vi "NF WF1973_74 SEQ Cst.vi"(8 "error in (no error)":errorcluster caption="Error IN", 10 "Ch(Ch1)":bool, 11 "VISAsession":refnum<visa-resource-name>) -> (0 "error out":errorcluster caption="Error OUT", 2 "Query Step":i32, 3 "CopyVISAsession":refnum<visa-resource-name>)   [LabVIEW 2010]
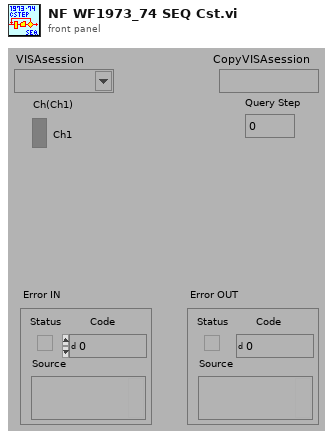
[diagram p1: front panel]
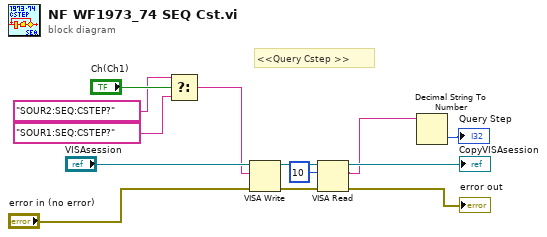
[diagram p0: block diagram]
diagram:
  # "<<Query Cstep >>"
  n1 = Select(t="SOUR2:SEQ:CSTEP?" ("文字列"), s="Ch(Ch1)", f="SOUR1:SEQ:CSTEP?" ("文字列")) -> (s? t:f=w3:string)
  n2 = VISA Write(VISA resource name="VISAsession", write buffer=w3, error in (no error)="error in (no error)") -> (VISA resource name out=w8:refnum<visa-resource-name>, error out=w9:errorcluster)  [unwired: 1 out]
  n3 = VISA Read(VISA resource name=w8, byte count=u32 10 ("バイトカウント（0）"), error in (no error)=w9) -> (VISA resource name out=→"CopyVISAsession":refnum<visa-resource-name>, read buffer=w1:string, error out=→"error out":errorcluster)  [unwired: 1 out]
  n4 = Decimal String To Number(string=w1) -> (number=→"Query Step":i32)  [unwired: 2 in, 1 out]
